vi "add_alignment_lines.vi"(7 "Color":u32(colorbox)=16448250, 11 "Image in":T1) -> (3 "Image out":T1)   [LabVIEW 2011]
uses:
  <vilib>/vision/Image Controls.llb/IMAQ Image.ctl
  global_vars.vi
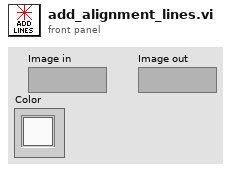
[diagram p1: front panel]
types:
  T1 = typedef "IMAQ Image.ctl" = refnum<image>
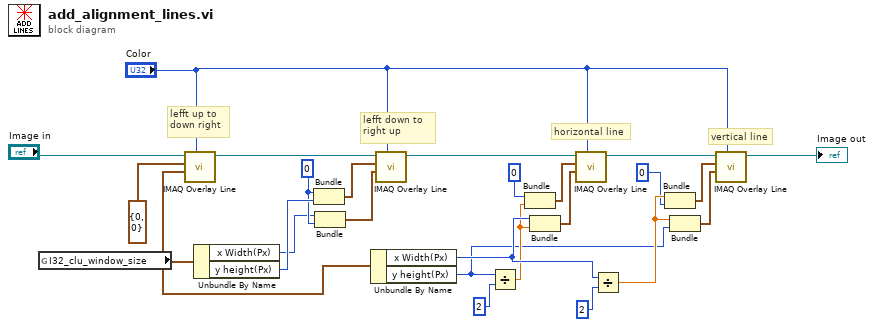
[diagram p0: block diagram]
diagram:
  w20 = 0 ("Y")
  # "vertical line"
  # "horizontal line"
  # "lefft down to \nright up"
  # "lefft up to\ndown right"
  n1 = global read "global_vars.vi" "I32_clu_window_size"() -> (w13:cluster{"x Width(Px)":i32, "y height(Px)":i32})
  n2 = call "IMAQ Overlay Line"("Color"="Color", "End Point"=w13, "Start Point"=cluster{"X":i32, "Y":i32} {"X"=0, "Y"=0}, "Image"="Image in") -> ("Image Out"=w21:T1)  [unwired: 6 in, 1 out]
  n3 = Unbundle By Name(w13) -> ("x Width(Px)"=w19:i32, "y height(Px)"=w23:i32)
  n4 = Bundle("Y"=w20, "y height(Px)"=w23) -> (w22:cluster{"Y":i32, "y height(Px)":i32})  [unwired: 1 in]
  n5 = Bundle("x Width(Px)"=w19, "Y"=w20) -> (w18:cluster{"x Width(Px)":i32, "Y":i32})  [unwired: 1 in]
  n6 = Unbundle By Name(w13) -> ("x Width(Px)"=w8:i32, "y height(Px)"=w2:i32)
  n7 = call "IMAQ Overlay Line"("Color"="Color", "End Point"=w18, "Start Point"=w22, "Image"=w21) -> ("Image Out"=w14:T1)  [unwired: 6 in, 1 out]
  n8 = Divide(x=w2, y=2) -> (x/y=w3:dbl)
  n9 = Bundle("Y"=0, w3) -> (w16:cluster{"Y":i32, dbl})  [unwired: 1 in]
  n10 = Bundle("x Width(Px)"=w8, w3) -> (w15:cluster{"x Width(Px)":i32, dbl})  [unwired: 1 in]
  n11 = call "IMAQ Overlay Line"("Color"="Color", "End Point"=w15, "Start Point"=w16, "Image"=w14) -> ("Image Out"=w7:T1)  [unwired: 6 in, 1 out]
  n12 = Divide(x=w8, y=2) -> (x/y=w5:dbl)
  n13 = Bundle(w5, "Y"=0) -> (w10:cluster{dbl, "Y":i32})  [unwired: 1 in]
  n14 = Bundle(w5, "y height(Px)"=w2) -> (w11:cluster{dbl, "y height(Px)":i32})  [unwired: 1 in]
  n15 = call "IMAQ Overlay Line"("Color"="Color", "End Point"=w11, "Start Point"=w10, "Image"=w7) -> ("Image Out"=→"Image out":T1)  [unwired: 6 in, 1 out]
